vi "ExcuseNotes_Panel.vi"(8 "error in (no error)":errorcluster, 11 "PanelController":refnum<class "MemberPanel.lvclass">) -> (0 "error out":errorcluster, 3 "ExcuseNotes.lvclass Out":refnum<class "ExcuseNotesHandler.lvclass">)   [LabVIEW 2015, in "Admin_Actor.lvlib"]
uses:
  Admin_Actor.lvlib
  ExcuseNotes/ExcuseNotesHandler.lvclass
  Member_Actor/MemberPanel/MemberPanel.lvclass
  ExcuseNotes/Type Definitions/Main Ctls And VI Refs.ctl
  Models/ListSelection/ListSelection.lvclass
  ExcuseNotes/ExcuseNotesHandler.lvclass/ExcuseNotesHandler.ctl
  <vilib>/Utility/error.llb/Error Cluster From Error Code.vi
  <vilib>/Utility/inputDevices.llb/mouseAcquire.vi
  <vilib>/ErrorRing/Error Ring.xnode
panel:
  in  "Commit":bool
  in  "SelectAll":bool
  in  "是否同意":bool
  in  "Name":string(combo)
  in  "Stop":bool
  in  "Table Control":string[][](table)
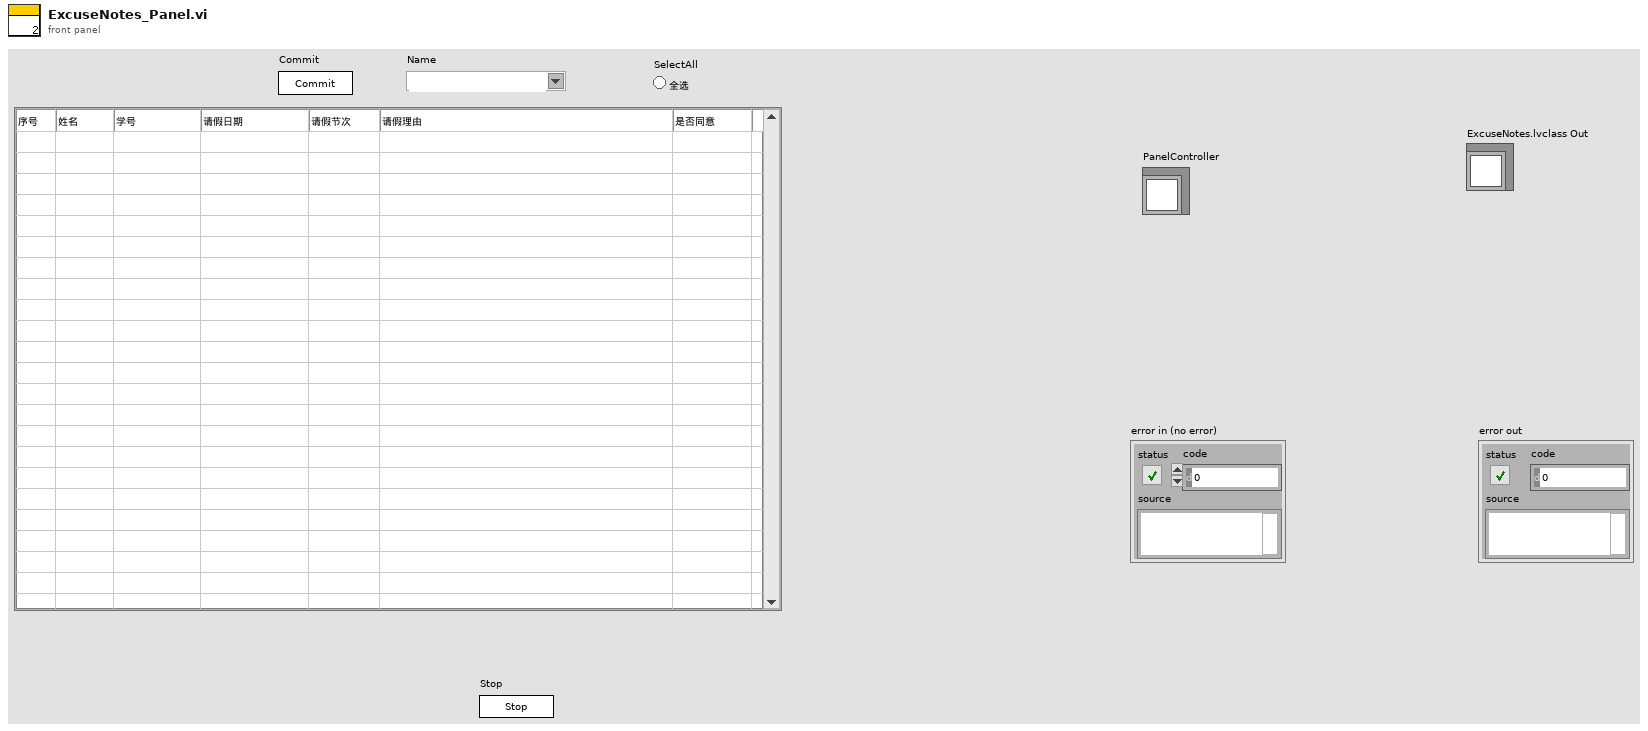
[diagram p1: front panel]
types:
  T1 = typedef "ExcuseNotesHandler.lvclass/Main Ctls And VI Refs.ctl" = cluster{"Table Control":refnum<vi>, "Stop":refnum<vi>, "是否同意":refnum<vi>, "Name":refnum<vi>, "全选":refnum<vi>, "VI Refnum":refnum<vi>}
  T2 = enum32{"Invalid", "Standard", "Closed", "Hidden", "Minimized", "Maximized"}
  T3 = cluster{"Horizontal":i32, "Vertical":i32, "Scrolling":i32}
  T4 = typedef "LVBoundsTypeDef.ctl" = cluster{"Width":u32, "Height":u32}
  T5 = typedef "LVPositionTypeDef.ctl" = cluster{"Left":i32, "Top":i32}
  T6 = typedef "LVPoint32TypeDef.ctl" = cluster{"Horizontal":i32, "Vertical":i32}
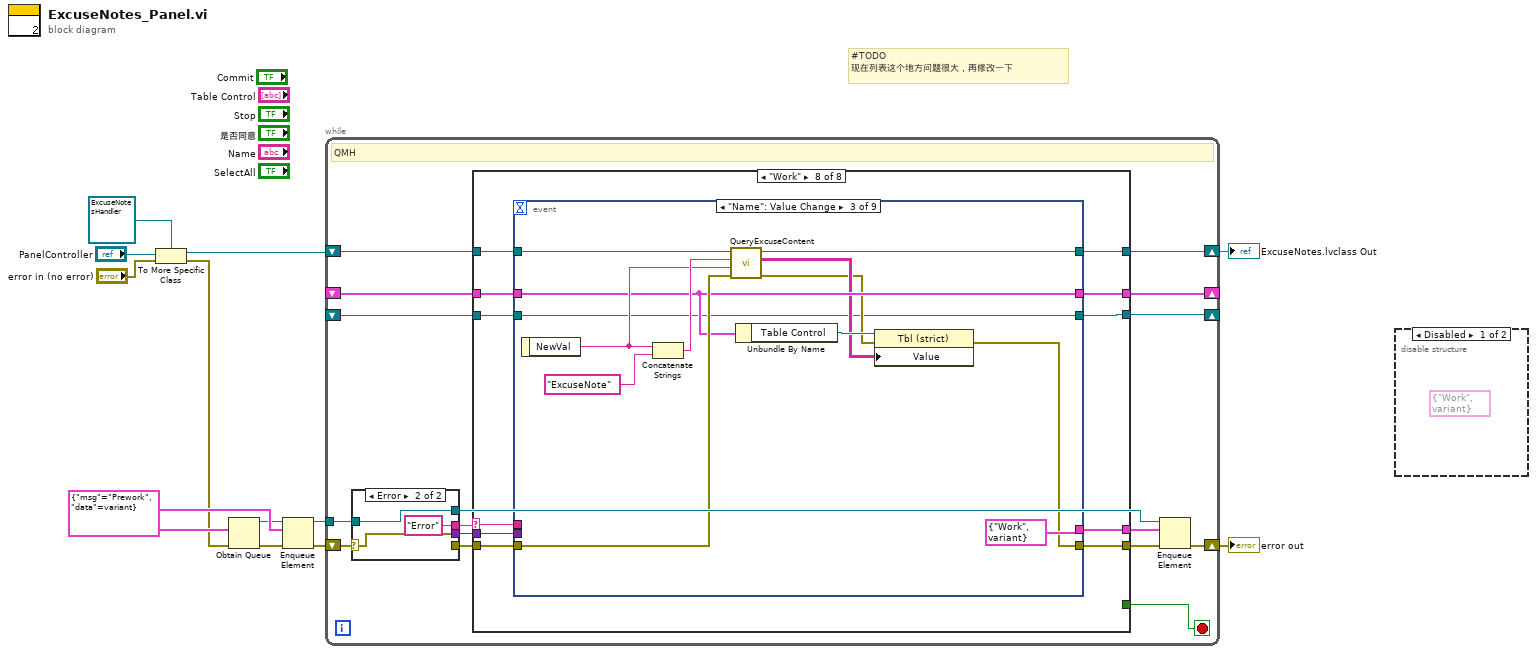
[diagram p0: block diagram]
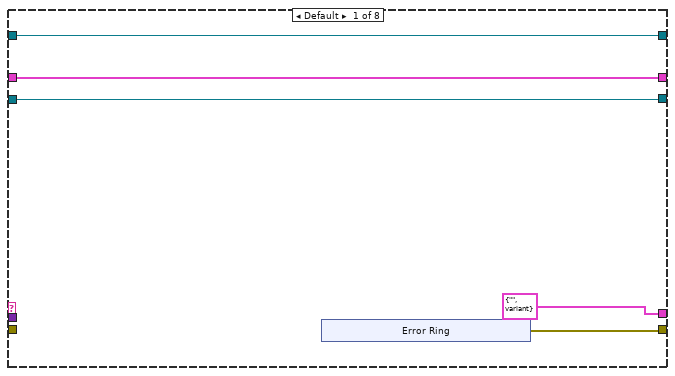
[diagram p3: hidden frame]
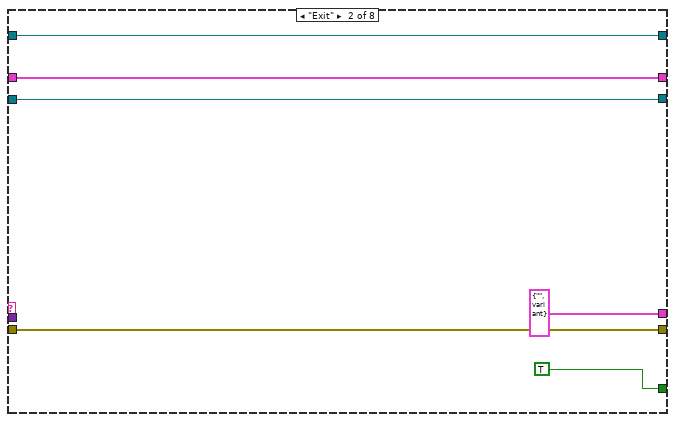
[diagram p4: hidden frame]
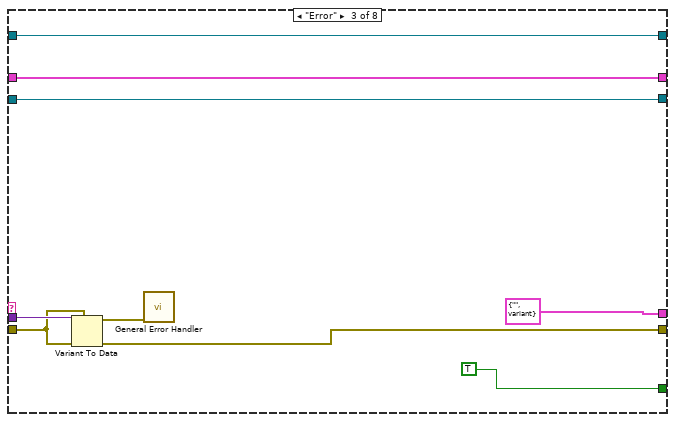
[diagram p5: hidden frame]
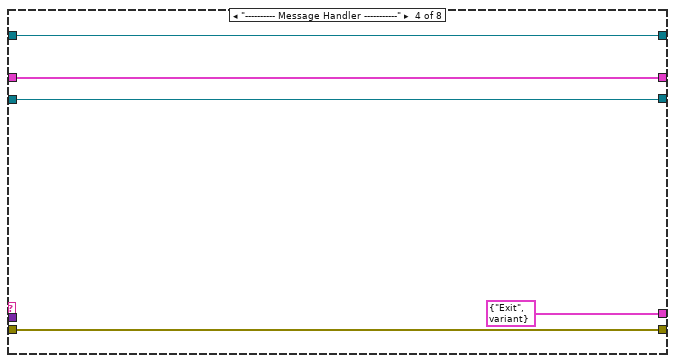
[diagram p6: hidden frame]
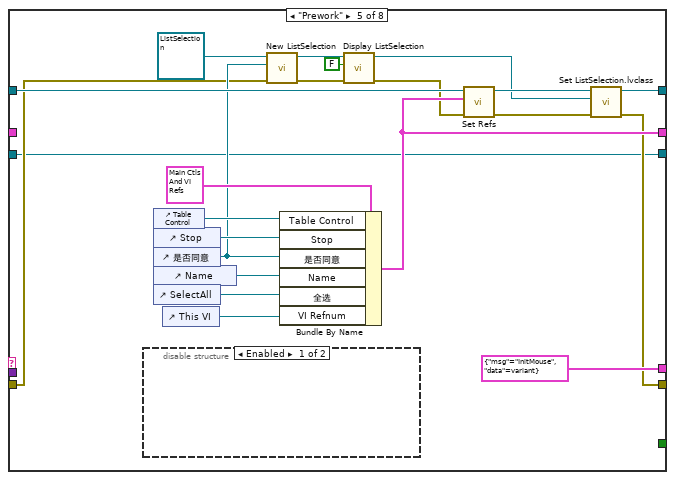
[diagram p7: hidden frame]
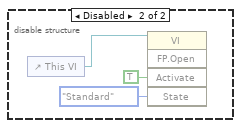
[diagram p8: hidden frame]
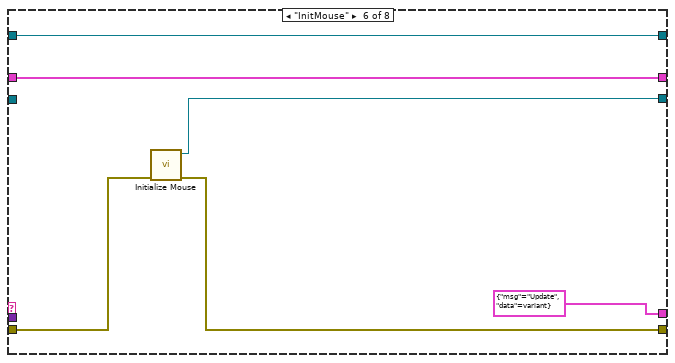
[diagram p9: hidden frame]
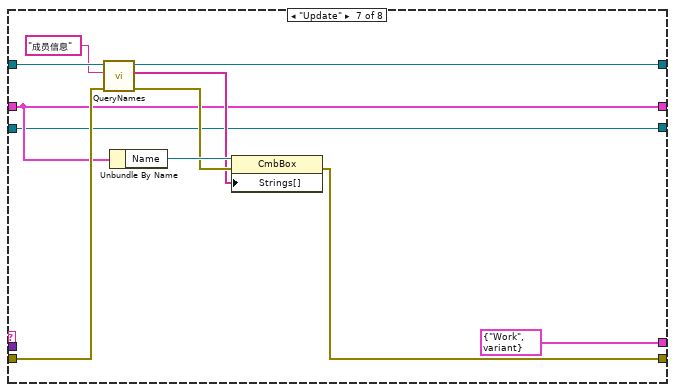
[diagram p10: hidden frame]
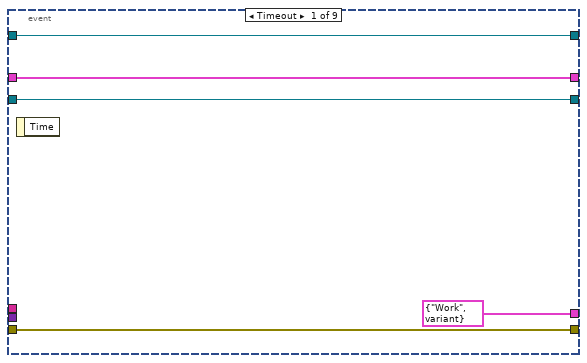
[diagram p11: hidden frame]
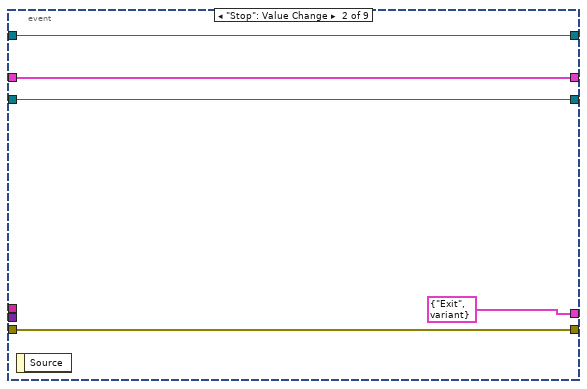
[diagram p12: hidden frame]
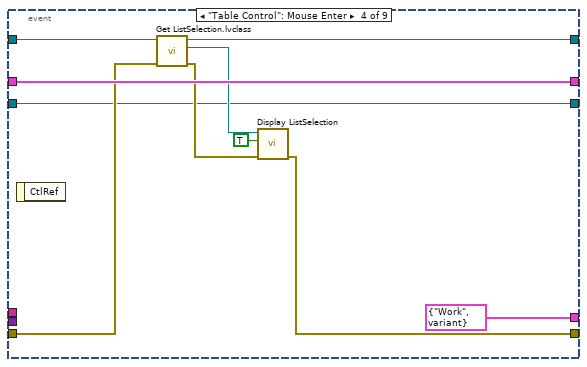
[diagram p13: hidden frame]
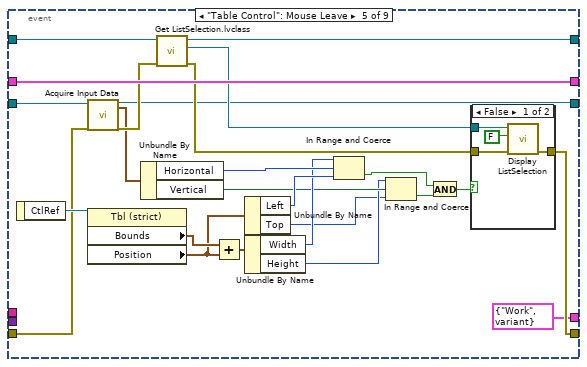
[diagram p14: hidden frame]
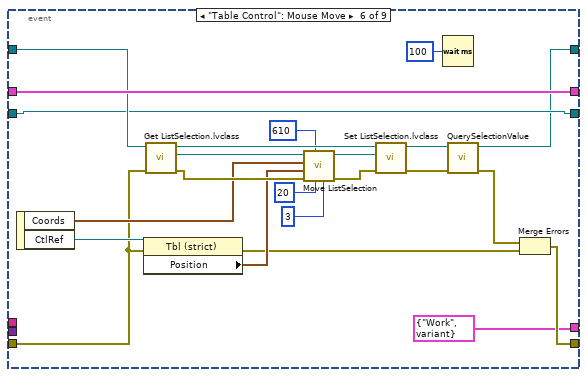
[diagram p16: hidden frame]
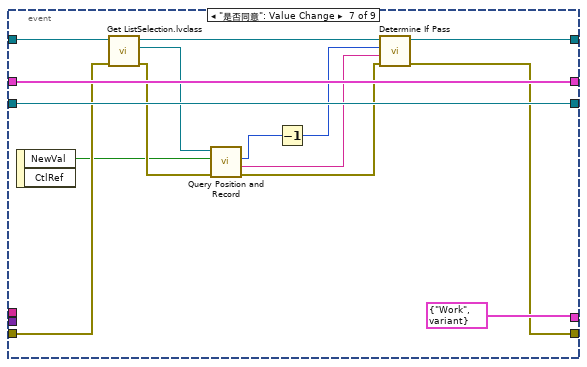
[diagram p17: hidden frame]
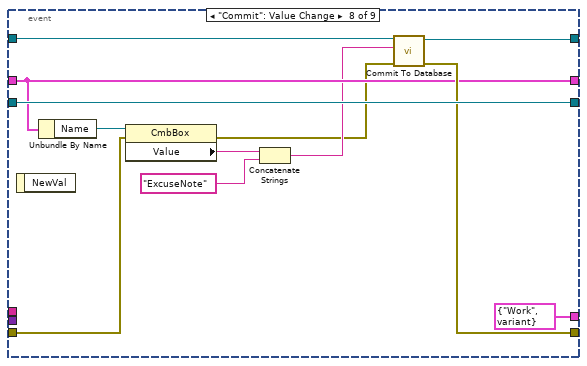
[diagram p18: hidden frame]
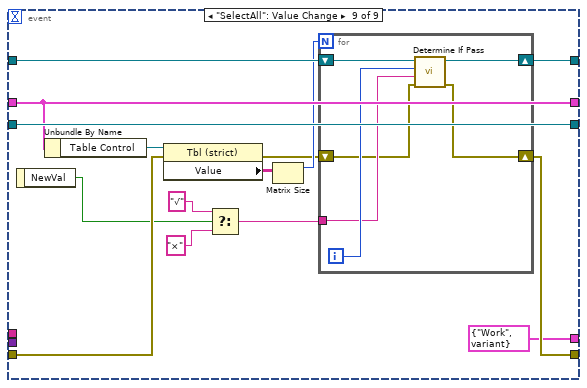
[diagram p19: hidden frame]
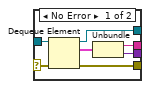
[diagram p20: hidden frame]
diagram:
  w10 = cluster{"msg":string, "data":variant} {"msg"="Prework", "data"=variant}
  # "#TODO \n现在列表这个地方问题很大，再修改一下"
  n1 = To More Specific Class(target class=refnum<class "ExcuseNotesHandler.lvclass"> refnum ("PanelController"), reference="PanelController", error in="error in (no error)") -> (specific class reference=w3:refnum<class "ExcuseNotesHandler.lvclass">, error out=w1:errorcluster)
  n2 = Obtain Queue(element data type=w10, error in (no error)=w1) -> (queue out=w8:refnum<queue>, error out=w9:errorcluster)  [unwired: 3 in, 1 out]
  n3 = Enqueue Element(queue=w8, element=w10, error in (no error)=w9) -> (queue out=w11:refnum<queue>, error out=w12:errorcluster)  [unwired: 1 in, 1 out]
  n4 = while {
    tunnel: w11 -> [w27]
    shift-right: [w22] -> w6
    shift-left: w12 -> [w28]
    shift-right: [w17] -> w7
    shift-left: w3 -> [w18]
    shift-right: [w16] -> _
    shift-left: _ -> [w15]
    shift-right: [w14] -> _
    shift-left: _ -> [w13]
    stop <- w19 stop-if-true
    # "QMH"
    n5 = case shown="Error" w28 {
      selector: w28 -> [w251 w255]
      tunnel: w27 -> [w252 w253]
      tunnel: [w250 _] -> w26
      tunnel: [w248 "Error" ("msg")] -> w25
      tunnel: [w247 w255] -> w24
      tunnel: [w246 w253] -> w21
      frame No Error {
        n6 = Dequeue Element(queue=w252, error in (no error)=w251) -> (queue out=w246:refnum<queue>, element=w249:cluster{"msg":string, "data":variant}, error out=w250:errorcluster)  [unwired: 1 in, 1 out]
        n7 = Unbundle(w249) -> ("msg"=w248:string, "data"=w247:variant)
      }
      frame Error {
      }
    }
    n8 = case shown="\"Work\"" w25 {
      selector: w25 -> [_ _ _ _ _ _ _ w109]
      tunnel: w26 -> [_ w44 w52 w58 w65 w86 w99 w111]
      tunnel: w24 -> [_ _ w53 _ _ _ _ w110]
      tunnel: [w33 w44 w50 w58 w69 w85 w92 w108] -> w23
      tunnel: [cluster{"msg":string, "data":variant} {"msg"="", "data"=variant} cluster{"msg":string, "data":variant} {"msg"="", "data"=variant} cluster{"msg":string, "data":variant} {"msg"="", "data"=variant} cluster{"msg":string, "data":variant} {"msg"="Exit", "data"=variant} cluster{"msg":string, "data":variant} {"msg"="InitMouse", "data"=variant} cluster{"msg":string, "data":variant} {"msg"="Update", "data"=variant} cluster{"msg":string, "data":variant} {"msg"="Work", "data"=variant} w107] -> w20
      tunnel: [_ TRUE TRUE _ _ _ _ _] -> w19
      tunnel: w18 -> [w31 w41 w47 w56 w73 w89 w100 w106]
      tunnel: [w31 w41 w47 w56 w68 w89 w94 w104] -> w17
      tunnel: [w30 w40 w46 w55 w72 w88 w93 w103] -> w16
      tunnel: w15 -> [w30 w40 w46 w55 _ w88 w93 w105]
      tunnel: [w29 w39 w45 w54 w59 w84 w90 w101] -> w14
      tunnel: w13 -> [w29 w39 w45 w54 w59 _ w90 w102]
      frame Default {
        n9 = xnode ("Error Ring")() -> ("error out"=w33:errorcluster)
      }
      frame "Exit" {
      }
      frame "Error" {
        n10 = Variant To Data(error in=w52, type=w52, Variant=w53) -> (data=w51:errorcluster, error out=w50:errorcluster)
        n11 = call <vilib>:"General Error Handler.vi"("error in (no error)"=w51) -> ()  [unwired: 10 in, 5 out]
      }
      frame "---------- Message Handler -----------" {
      }
      frame "Prework" {
        n12 = disable-structure shown="Enabled" {
          frame Enabled {
          }
          frame Disabled {
            n13 = control-ref of="This VI"() -> (w83:refnum<vi>)
            n14 = invoke class="VI" method="FP.Open"(reference=w83, "Activate"=TRUE ("Activate?"), "State"=T2."Standard") -> ()  [unwired: 2 in, 5 out]
          }
        }
        n15 = control-ref of="Table Control"() -> (w78:refnum<vi>)
        n16 = control-ref of="Stop"() -> (w77:refnum<vi>)
        n17 = control-ref of="是否同意"() -> (w66:refnum<vi>)
        n18 = control-ref of="Name"() -> (w76:refnum<vi>)
        n19 = control-ref of="SelectAll"() -> (w75:refnum<vi>)
        n20 = control-ref of="This VI"() -> (w74:refnum<vi>)
        n21 = call "New ListSelection.vi"("error in (no error)"=w65, "Bool Refnum"=w66, "ListSelection in"=refnum<class "ListSelection.lvclass"> refnum ("Admin_Actor.lvlib:ListSelection.lvclass")) -> ("error out"=w63:errorcluster, "ListSelection out"=w64:refnum<class "ListSelection.lvclass">)  [unwired: 7 in]
        n22 = Bundle By Name(cluster=T1 {"Table Control"=refnum, "Stop"=refnum, "是否同意"=refnum, "Name"=refnum, "全选"=refnum, "VI Refnum"=refnum} ("Refs"), "Table Control"=w78, "Stop"=w77, "是否同意"=w66, "Name"=w76, "全选"=w75, "VI Refnum"=w74) -> (w72:T1)
        n23 = call "Display ListSelection.vi"("error in (no error)"=w63, "Visible(False)"=FALSE, "ListSelection in"=w64) -> ("error out"=w61:errorcluster, "ListSelection out"=w62:refnum<class "ListSelection.lvclass">)  [unwired: 7 in]
        n24 = call "Set Refs.vi"("error in (no error)"=w61, "Refs"=w72, "ExcuseNotes in"=w73) -> ("error out"=w70:errorcluster, "ExcuseNotes out"=w71:refnum<class "ExcuseNotesHandler.lvclass">)  [unwired: 7 in]
        n25 = call "Set ListSelection.lvclass.vi"("error in (no error)"=w70, "Admin_Actor.lvlib:ListSelection.lvclass"=w62, "ExcuseNotesHandler in"=w71) -> ("error out"=w69:errorcluster, "ExcuseNotesHandler out"=w68:refnum<class "ExcuseNotesHandler.lvclass">)  [unwired: 7 in]
      }
      frame "InitMouse" {
        n26 = call <vilib>:"Initialize Mouse.vi"("error in (no error)"=w86) -> ("error out"=w85:errorcluster, "device ID"=w84:refnum<k1>)  [unwired: 9 in]
      }
      frame "Update" {
        n27 = call "QueryNames.vi"("error in (no error)"=w99, "TableName(\"\")"="成员信息" ("TableName(\"\")"), "ExcuseNotes in"=w100) -> ("error out"=w96:errorcluster, "Names(\"\")"=w95:string[], "ExcuseNotes out"=w94:refnum<class "ExcuseNotesHandler.lvclass">)  [unwired: 6 in]
        n28 = Unbundle By Name(w93) -> ("Name"=w97:refnum<vi>)
        n29 = property class="CmbBox"(reference=w97, error in=w96, "Strings[]"=w95) -> (error out=w92:errorcluster)  [unwired: 1 out]
      }
      frame "Work" {
        n30 = event shown="[2] \"Name\": Value Change" {
          selector: _ -> [_ _ _ _ _ _ _ _ _]
          dyn-events: _ -> [_ _ _ _ _ _ _ _ _]
          timeout: _ -> [_ _ _ _ _ _ _ _ _]
          tunnel: w111 -> [w116 w121 w132 w142 w159 w188 w206 w217 w235]
          tunnel: w110 -> [_ _ _ _ _ _ _ _ _]
          tunnel: w109 -> [_ _ _ _ _ _ _ _ _]
          tunnel: [w116 w121 w123 w138 w165 w183 w209 w221 w226] -> w108
          tunnel: [cluster{"msg":string, "data":variant} {"msg"="Work", "data"=variant} cluster{"msg":string, "data":variant} {"msg"="Exit", "data"=variant} cluster{"msg":string, "data":variant} {"msg"="Work", "data"=variant} cluster{"msg":string, "data":variant} {"msg"="Work", "data"=variant} cluster{"msg":string, "data":variant} {"msg"="Work", "data"=variant} cluster{"msg":string, "data":variant} {"msg"="Work", "data"=variant} cluster{"msg":string, "data":variant} {"msg"="Work", "data"=variant} cluster{"msg":string, "data":variant} {"msg"="Work", "data"=variant} cluster{"msg":string, "data":variant} {"msg"="Work", "data"=variant}] -> w107
          tunnel: w106 -> [w114 w119 w133 w143 w168 w196 w207 w223 w238]
          tunnel: w105 -> [w113 w118 w127 w144 w169 w197 w212 w219 w237]
          tunnel: [w114 w119 w128 w136 w163 w176 w208 w222 w227] -> w104
          tunnel: [w113 w118 w127 w144 w169 w197 w212 w219 w237] -> w103
          tunnel: w102 -> [w112 w117 w122 w135 w160 w180 w210 w224 w239]
          tunnel: [w112 w117 w122 w135 w157 w180 w210 w224 w239] -> w101
          event Timeout {
            n31 = event-data() -> ()  [unwired: 1 in, 1 out]
          }
          event "Stop": Value Change {
            n32 = event-data() -> ()  [unwired: 1 in, 1 out]
          }
          event "Name": Value Change {
            n33 = event-data() -> ("NewVal"=w130:string)  [unwired: 1 in]
            n34 = Concatenate Strings(w130, "ExcuseNote" ("string")) -> (w131:string)
            n35 = call "QueryExcuseContent.vi"("error in (no error)"=w132, "Name"=w130, "TableName"=w131, "ExcuseNotesHandler"=w133) -> ("error out"=w124:errorcluster, "ExcuseNote(\"\")"=w125:string[][], "ExcuseNotesHandler Out"=w128:refnum<class "ExcuseNotesHandler.lvclass">)  [unwired: 5 in]
            n36 = Unbundle By Name(w127) -> ("Table Control"=w126:refnum<vi>)
            n37 = property class="Tbl (strict)"(reference=w126, error in=w124, "Value"=w125) -> (error out=w123:errorcluster)  [unwired: 1 out]
          }
          event "Table Control": Mouse Enter {
            n38 = event-data() -> ()  [unwired: 1 in, 1 out]
            n39 = call "Get ListSelection.lvclass.vi"("error in (no error)"=w142, "ExcuseNotesHandler in"=w143) -> ("error out"=w140:errorcluster, "Admin_Actor.lvlib:ListSelection.lvclass"=w141:refnum<class "ListSelection.lvclass">, "ExcuseNotesHandler out"=w136:refnum<class "ExcuseNotesHandler.lvclass">)  [unwired: 7 in]
            n40 = call "Display ListSelection.vi"("error in (no error)"=w140, "Visible(False)"=TRUE, "ListSelection in"=w141) -> ("error out"=w138:errorcluster)  [unwired: 7 in, 1 out]
          }
          event "Table Control": Mouse Leave {
            n41 = event-data() -> ("CtlRef"=w162:refnum<vi>)  [unwired: 1 in]
            n42 = call-poly <vilib>:"Acquire Input Data.vi"("device ID"=w160, "error in (no error)"=w159) -> ("device ID"=w157:refnum<k1>, "axis info"=w156:T3, "error out"=w158:errorcluster)  [unwired: 14 in, 1 out]
            n43 = property class="Tbl (strict)"(reference=w162) -> ("Bounds"=w161:T4, "Position"=w155:T5)  [unwired: 1 in, 2 out]
            n44 = Unbundle By Name(w156) -> ("Horizontal"=w153:i32, "Vertical"=w150:i32)
            n45 = call "Get ListSelection.lvclass.vi"("error in (no error)"=w158, "ExcuseNotesHandler in"=w168) -> ("error out"=w166:errorcluster, "Admin_Actor.lvlib:ListSelection.lvclass"=w167:refnum<class "ListSelection.lvclass">, "ExcuseNotesHandler out"=w163:refnum<class "ExcuseNotesHandler.lvclass">)  [unwired: 7 in]
            n46 = Add(x=w161, y=w155) -> (x+y=w154:T4)
            n47 = Unbundle By Name(w155) -> ("Left"=w152:i32, "Top"=w148:i32)
            n48 = Unbundle By Name(w154) -> ("Width"=w151:u32, "Height"=w149:u32)
            n49 = In Range and Coerce(upper limit=w151, x=w153, lower limit=w152) -> (In Range?=w147:bool)  [unwired: 1 out]
            n50 = In Range and Coerce(upper limit=w149, x=w150, lower limit=w148) -> (In Range?=w146:bool)  [unwired: 1 out]
            n51 = And(x=w147, y=w146) -> (x .and. y?=w145:bool)
            n52 = case shown="False" w145 {
              tunnel: w167 -> [w173 _]
              tunnel: w166 -> [w172 w174]
              tunnel: [w170 w174] -> w165
              frame False {
                n53 = call "Display ListSelection.vi"("error in (no error)"=w172, "Visible(False)"=FALSE, "ListSelection in"=w173) -> ("error out"=w170:errorcluster)  [unwired: 7 in, 1 out]
              }
              frame True {
              }
            }
          }
          event "Table Control": Mouse Move {
            n54 = event-data() -> ("Coords"=w190:T6, "CtlRef"=w189:refnum<vi>)  [unwired: 1 in]
            n55 = property class="Tbl (strict)"(reference=w189, error in=w188) -> (error out=w184:errorcluster, "Position"=w187:T5)  [unwired: 1 out]
            n56 = call "Get ListSelection.lvclass.vi"("error in (no error)"=w188, "ExcuseNotesHandler in"=w196) -> ("error out"=w192:errorcluster, "Admin_Actor.lvlib:ListSelection.lvclass"=w195:refnum<class "ListSelection.lvclass">, "ExcuseNotesHandler out"=w194:refnum<class "ExcuseNotesHandler.lvclass">)  [unwired: 7 in]
            n57 = call "Move ListSelection.vi"("Bias"=3, "Size"=20, "Herizon"=610 ("Size"), "error in (no error)"=w192, "List_Rec"=w187, "Mou_Pos"=w190, "ListSelection in"=w195) -> ("error out"=w191:errorcluster, "ListSelection out"=w193:refnum<class "ListSelection.lvclass">)  [unwired: 3 in]
            n58 = call "Set ListSelection.lvclass.vi"("error in (no error)"=w191, "Admin_Actor.lvlib:ListSelection.lvclass"=w193, "ExcuseNotesHandler in"=w194) -> ("error out"=w178:errorcluster, "ExcuseNotesHandler out"=w179:refnum<class "ExcuseNotesHandler.lvclass">)  [unwired: 7 in]
            n59 = Wait (ms)(milliseconds to wait=u32 100) -> ()  [unwired: 1 out]
            n60 = call "QuerySelectionValue.vi"("error in (no error)"=w178, "ExcuseNotesHandler in"=w179) -> ("error out"=w177:errorcluster, "ExcuseNotesHandler out"=w176:refnum<class "ExcuseNotesHandler.lvclass">)  [unwired: 8 in]
            n61 = Merge Errors(w177, w184) -> (w183:errorcluster)
          }
          event "是否同意": Value Change {
            n62 = event-data() -> ("NewVal"=w203:bool)  [unwired: 1 in, 1 out]
            n63 = call "Get ListSelection.lvclass.vi"("error in (no error)"=w206, "ExcuseNotesHandler in"=w207) -> ("error out"=w204:errorcluster, "Admin_Actor.lvlib:ListSelection.lvclass"=w205:refnum<class "ListSelection.lvclass">, "ExcuseNotesHandler out"=w202:refnum<class "ExcuseNotesHandler.lvclass">)  [unwired: 7 in]
            n64 = call "Query Position and Record.vi"("error in (no error)"=w204, "SelectKey(True)"=w203, "ListSelection in"=w205) -> ("error out"=w200:errorcluster, "SignedResult(\"\")"=w201:string, "InxOfColumns"=w199:i32)  [unwired: 5 in, 1 out]
            n65 = Decrement(x=w199) -> (x-1=w198:i32)
            n66 = call "Determine If Pass.vi"("error in (no error)"=w200, "DetermineResult(\"\")"=w201, "SelectRow(0)"=w198, "ExcuseNotesHandler in"=w202) -> ("error out"=w209:errorcluster, "ExcuseNotesHandler out"=w208:refnum<class "ExcuseNotesHandler.lvclass">)  [unwired: 6 in]
          }
          event "Commit": Value Change {
            n67 = event-data() -> ()  [unwired: 1 in, 1 out]
            n68 = Unbundle By Name(w219) -> ("Name"=w218:refnum<vi>)
            n69 = property class="CmbBox"(reference=w218, error in=w217) -> (error out=w213:errorcluster, "Value"=w216:string)  [unwired: 1 out]
            n70 = Concatenate Strings(w216, "ExcuseNote" ("string")) -> (w214:string)
            n71 = call "Commit To Database.vi"("error in (no error)"=w213, "TableName(\"\")"=w214, "ExcuseNotesHandler in"=w223) -> ("error out"=w221:errorcluster, "ExcuseNotesHandler out"=w222:refnum<class "ExcuseNotesHandler.lvclass">)  [unwired: 7 in]
          }
          event "SelectAll": Value Change {
            n72 = event-data() -> ("NewVal"=w232:bool)  [unwired: 1 in]
            n73 = Unbundle By Name(w237) -> ("Table Control"=w236:refnum<vi>)
            n74 = property class="Tbl (strict)"(reference=w236, error in=w235) -> (error out=w228:errorcluster, "Value"=w234:string[][])  [unwired: 1 out]
            n75 = Select(t="√", s=w232, f="×") -> (s? t:f=w229:string)
            n76 = Matrix Size(0:w234) -> (1:w233:i32)  [unwired: 1 out]
            n77 = for {
              N: w233 -> [_]
              tunnel: w229 -> [w243]
              shift-right: [w241] -> w227
              shift-left: w238 -> [w245]
              shift-right: [w240] -> w226
              shift-left: w228 -> [w242]
              i -> [w244]
              n78 = call "Determine If Pass.vi"("error in (no error)"=w242, "DetermineResult(\"\")"=w243, "SelectRow(0)"=w244, "ExcuseNotesHandler in"=w245) -> ("error out"=w240:errorcluster, "ExcuseNotesHandler out"=w241:refnum<class "ExcuseNotesHandler.lvclass">)  [unwired: 6 in]
            }
          }
        }
      }
    }
    n79 = Enqueue Element(queue=w21, element=w20, error in (no error)=w23) -> (error out=w22:errorcluster)  [unwired: 1 in, 2 out]
  }
  "ExcuseNotes.lvclass Out" <- w7
  "error out" <- w6
  n80 = disable-structure shown="Disabled" {
    frame Disabled {
      (unwired) cluster{"msg":string, "data":variant} {"msg"="Work", "data"=variant}
    }
    frame Enabled {
    }
  }
